vi "数组的更多使用4，以及信号处理函数的使用.vi"() -> ()   [LabVIEW 2018]
uses:
  <vilib>/measure/NI_MABase.lvlib
  <vilib>/measure/NI_MAPro.lvlib
  <vilib>/measure/madcrms.llb/Basic Averaged DC-RMS for 1 Chan.vi
  <vilib>/express/express signal manip/GetorSetDDTAttributes/Get DDT Attributes/Get DDT Properties.xnode
  <vilib>/express/express signal manip/GetorSetDDTAttributes/Shared VIs/TimeType.ctl
  <vilib>/express/express signal manip/GetorSetDDTAttributes/Shared VIs/GetSetShared.lvlib
  <vilib>/express/express signal manip/GetorSetDDTAttributes/Shared VIs/XDimension.ctl
  <vilib>/measure/mascope.llb/Cycle Average and RMS 1 chan.vi
  <vilib>/measure/madcrms.llb/Averaged DC-RMS for 1 Chan.vi
  <vilib>/measure/mascope.llb/Transition Measurements 1 chan.vi
  <vilib>/measure/mascope.llb/Pulse Measurements 1 chan.vi
  <vilib>/measure/mascope.llb/Amplitude and Levels 1 chan.vi
  <vilib>/express/express shared/transition.llb/Dynamic To Waveform Array.vi
  <vilib>/express/express signal manip/GetorSetDDTAttributes/Shared VIs/XDimension conversion.vi
panel:
  in  "frequency 2":dbl=10.0 caption="频率" format="%0.2p"
  in  "等待时间（毫秒）":u32=600
  in  "布尔":bool
  out "波形图表 2":waveform(dbl)(graph)
  in  "信号索引":i32
  out "单位":string
  out "X维":T1
  out "起始时间标识":timestamp
  out "时间标识":timestamp
  out "时间模式":T2
  out "信号名称":string
  out "波形图":dynamicdata(graph)
  out "low state level":dbl caption="低状态电平" format="%.2g"
  out "high state level":dbl caption="高状态电平" format="%.2g"
  out "amplitude 2":dbl caption="幅值" format="%.2p"
  out "duty cycle":dbl caption="占空比" format="%.2g"
  out "pulse duration":dbl caption="脉冲持续期" format="%.2g"
  out "period":dbl caption="周期" format="%.2g"
  out "post-transition":T3 caption="后瞬态"
  out "pre-transition":T3 caption="前瞬态"
  out "transition duration":dbl caption="瞬态持续期"
  out "RMS value waveform":waveform(dbl) caption="均方根值波形"
  out "DC value waveform":waveform(dbl) caption="直流波形"
  out "cycle RMS":dbl caption="周期均方根" format="%.2g"
  out "cycle average":dbl caption="周期平均" format="%.2p"
  out "RMS value 2":dbl caption="均方根值" format="%0.2p"
  out "DC value 2":dbl caption="直流值" format="%0.2p"
  out "正弦":dynamicdata(graph)
  in  "Phase":dbl caption="相位"
  in  "Amplitude":dbl=1.0 caption="幅值"
  in  "Frequency":dbl=10.1 caption="频率"
  in  "Reset Signal":bool caption="重置信号"
  in  "Offset":dbl caption="偏移量"
  out "DC value":dbl caption="直流值" format="%0.2p"
  out "RMS value":dbl caption="均方根值" format="%0.2p"
  in  "frequency":dbl=10.0 caption="频率" format="%0.2p"
  in  "amplitude":dbl=1.0 caption="幅值" format="%0.2p"
  in  "phase":dbl caption="相位" format="%.2p"
  in  "signal type":T4(ring) caption="信号类型"
  in  "reset signal":bool caption="重置信号"
  in  "square wave duty cycle (%)":dbl=50.0 caption="方波占空比(%)" format="%0.2f"
  in  "offset":dbl caption="偏移量" format="%0.2p"
  out "波形图表":waveform(dbl)(graph)
  in  "枚举":enum16{"王五", "李四", "张三"}(ring)
  in  "下拉列表":u16(ring) items=["王五"=50, "李四"=40, "张三"=30]
  out "初始化的数组 2":bool[][](array[boolean])
  in  "维数大小 4":i32
  in  "维数大小 3":i32
  out "初始化的数组":dbl[][](array[numeric])
  in  "维数大小 2":i32
  in  "维数大小":i32
  in  "元素":dbl
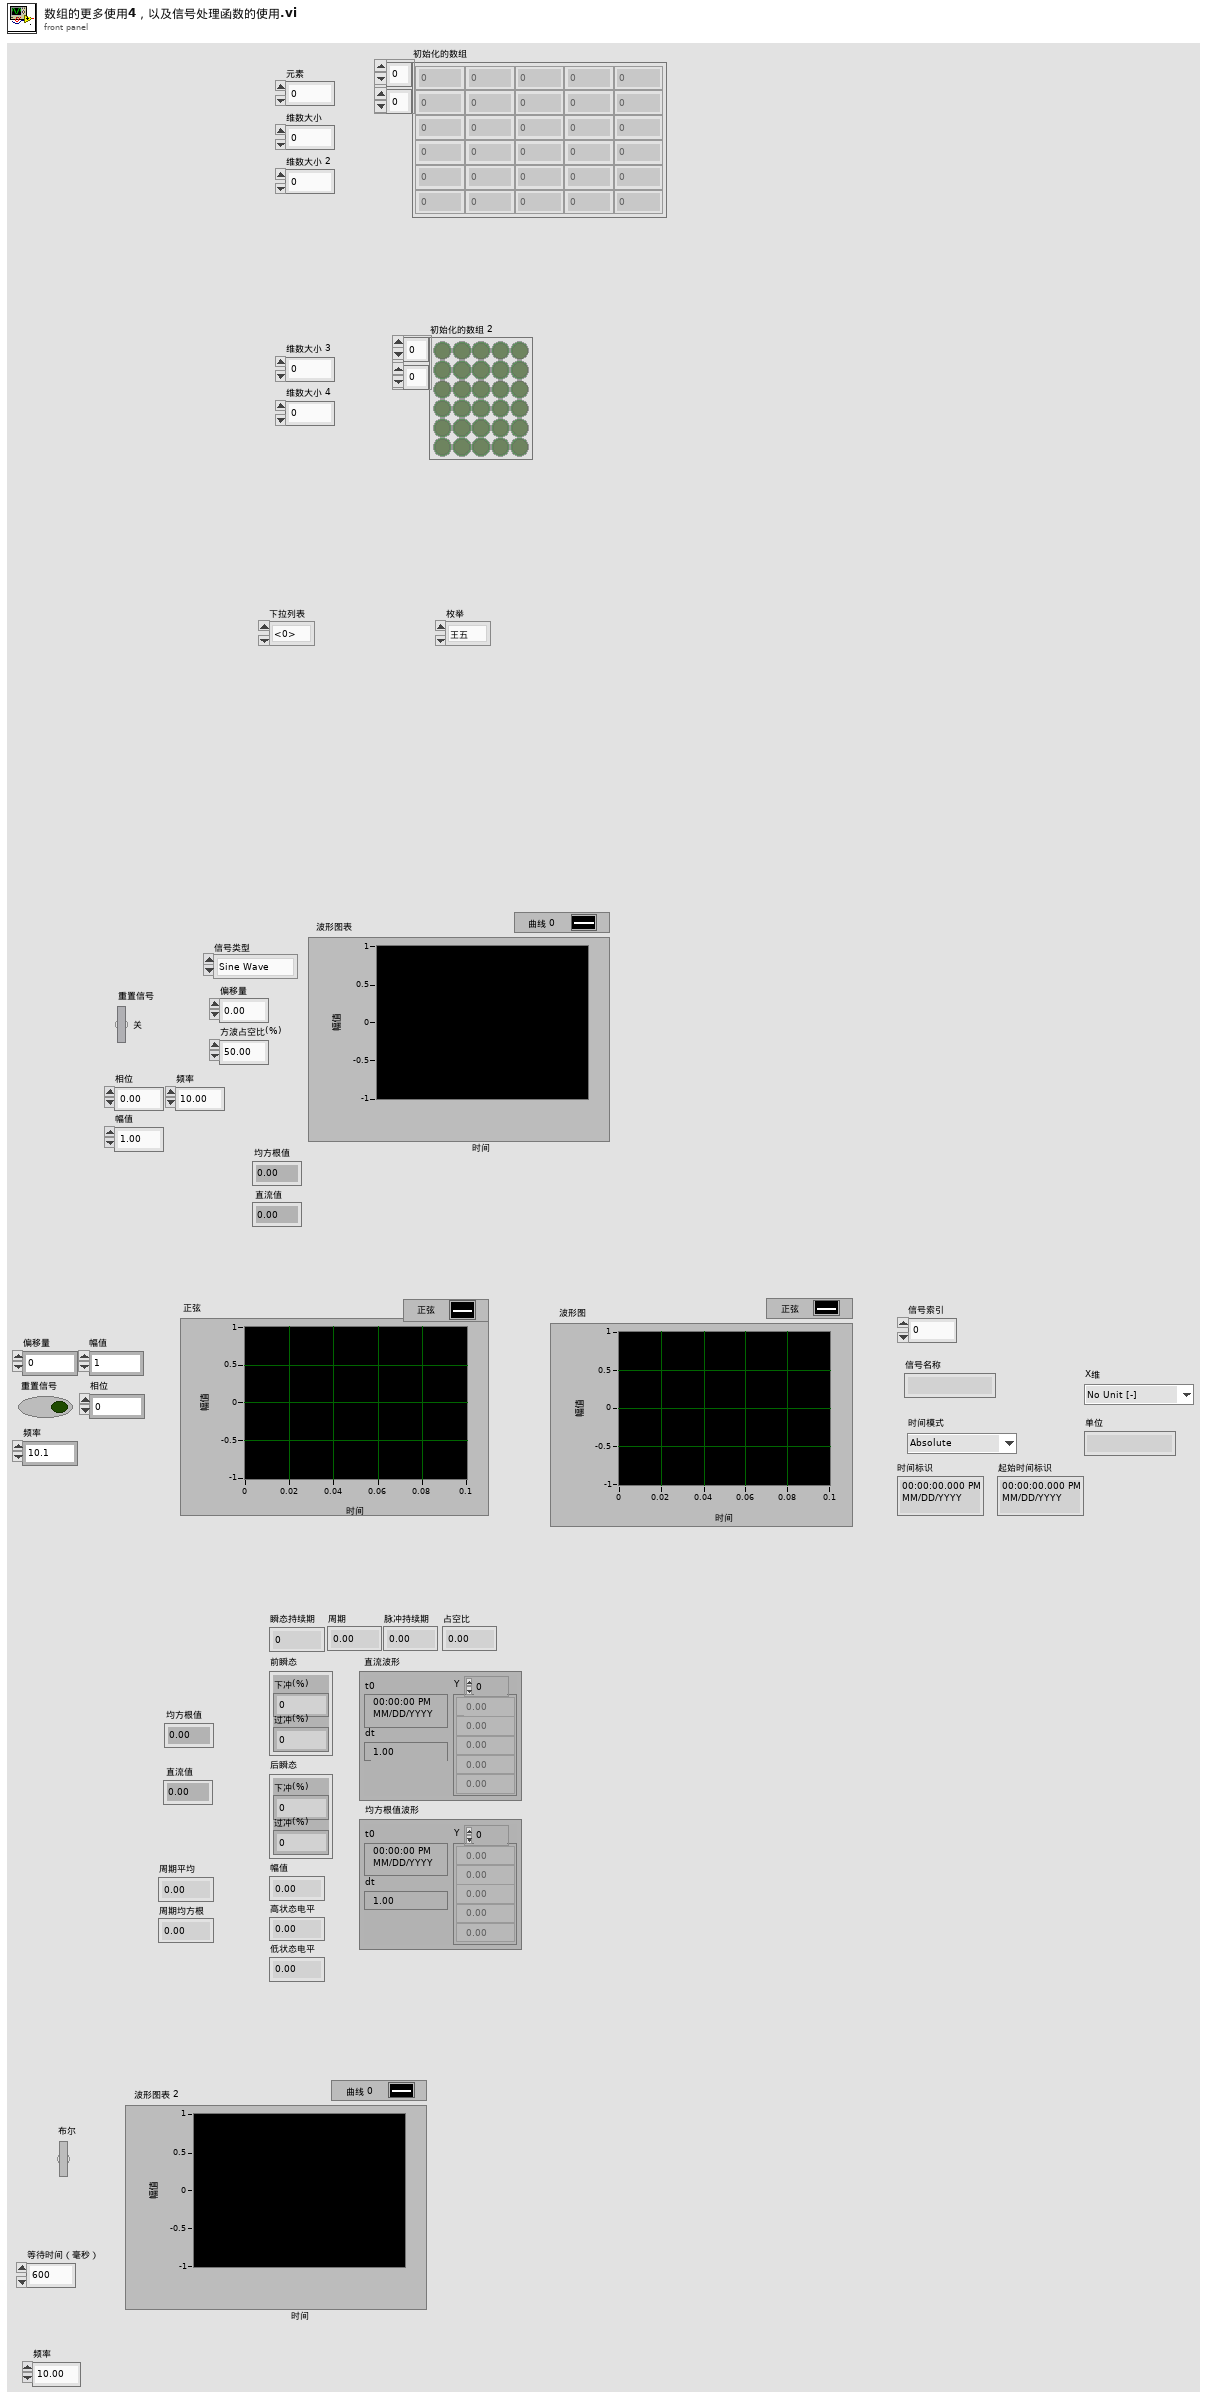
[diagram p1: front panel]
types:
  T1 = typedef "GetSetShared.lvlib/XDimension.ctl" = enum16{"No Unit [-]", "Time [sec]", "Frequency [Hz]"}
  T2 = typedef "GetSetShared.lvlib/TimeType.ctl" = enum16{"Absolute", "Relative"}
  T3 = cluster{"undershoot (%)":dbl, "overshoot (%)":dbl}
  T4 = enum16{"Sine Wave", "Triangle Wave", "Square Wave", "Sawtooth Wave"}
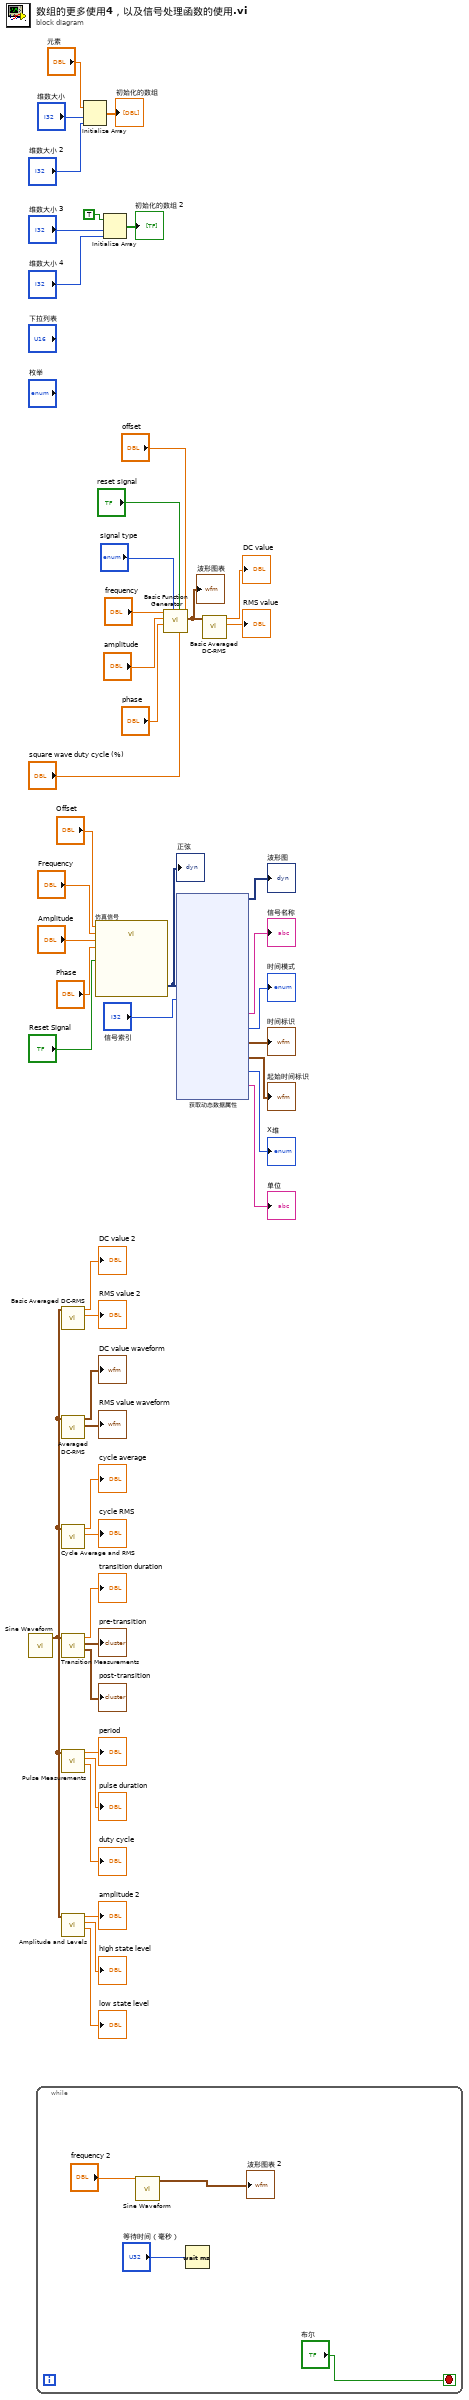
[diagram p0: block diagram]
diagram:
  n1 = call <vilib>:"Sine Waveform.vi"() -> ("signal out"=w9:waveform(dbl))  [unwired: 10 in, 1 out]
  n2 = while {
    stop <- "布尔" stop-if-true
    n3 = call <vilib>:"Sine Waveform.vi"("frequency"="frequency 2") -> ("signal out"=→"波形图表 2":waveform(dbl))  [unwired: 9 in, 1 out]
    n4 = Wait (ms)(milliseconds to wait="等待时间（毫秒）") -> ()  [unwired: 1 out]
  }
  n5 = call-poly <vilib>:"Basic Averaged DC-RMS.vi"("signal in"=w9) -> ("RMS value"=→"RMS value 2":dbl, "DC value"=→"DC value 2":dbl)  [unwired: 7 in, 2 out]
  n6 = call-poly <vilib>:"Averaged DC-RMS.vi"("signal in"=w9) -> ("RMS value waveform"=→"RMS value waveform":waveform(dbl), "DC value waveform"=→"DC value waveform":waveform(dbl))  [unwired: 6 in, 3 out]
  n7 = call-poly <vilib>:"Cycle Average and RMS.vi"("signal in"=w9) -> ("cycle RMS"=→"cycle RMS":dbl, "cycle average"=→"cycle average":dbl)  [unwired: 7 in, 2 out]
  n8 = call-poly <vilib>:"Transition Measurements.vi"("signal in"=w9) -> ("post-transition"=→"post-transition":T3, "pre-transition"=→"pre-transition":T3, "transition duration"=→"transition duration":dbl)  [unwired: 5 in, 3 out]
  n9 = call-poly <vilib>:"Pulse Measurements.vi"("signal in"=w9) -> ("duty cycle"=→"duty cycle":dbl, "pulse duration"=→"pulse duration":dbl, "period"=→"period":dbl)  [unwired: 6 in, 2 out]
  n10 = call-poly <vilib>:"Amplitude and Levels.vi"("signal in"=w9) -> ("low state level"=→"low state level":dbl, "high state level"=→"high state level":dbl, "amplitude"=→"amplitude 2":dbl)  [unwired: 7 in, 1 out]
  n11 = Initialize Array("元素", "维数大小", "维数大小 2") -> (→"初始化的数组":dbl[][])
  n12 = call "仿真信号"("Offset"="Offset", "Reset Signal"="Reset Signal", "Frequency"="Frequency", "Amplitude"="Amplitude", "Phase"="Phase") -> ("正弦"=w25:dynamicdata)  [unwired: 9 in, 1 out]
  "正弦" <- w25
  n13 = Initialize Array(TRUE, "维数大小 3", "维数大小 4") -> (→"初始化的数组 2":bool[][])
  n14 = call <vilib>:"Basic Function Generator.vi"("offset"="offset", "square wave duty cycle (%)"="square wave duty cycle (%)", "reset signal"="reset signal", "signal type"="signal type", "phase"="phase", "amplitude"="amplitude", "frequency"="frequency") -> ("signal out"=w33:waveform(dbl))  [unwired: 2 in, 2 out]
  "波形图表" <- w33
  n15 = xnode "获取动态数据属性"("信号输入"=w25, "信号索引"="信号索引") -> ("信号名称"=→"信号名称":string, "时间模式"=→"时间模式":T2, "时间标识"=→"时间标识":timestamp, "起始时间标识"=→"起始时间标识":timestamp, "X维"=→"X维":T1, "单位"=→"单位":string, "信号输出"=→"波形图":dynamicdata)  [unwired: 1 in, 1 out]
  n16 = call-poly <vilib>:"Basic Averaged DC-RMS.vi"("signal in"=w33) -> ("RMS value"=→"RMS value":dbl, "DC value"=→"DC value":dbl)  [unwired: 7 in, 2 out]
